vi "Close Session.vi"(8 "error in (no error)":errorcluster, 11 "VISA resource name":refnum<visa-resource-name>) -> ()   [LabVIEW 2014]
panel:
  in  "Reset? (T: Yes)":bool=TRUE
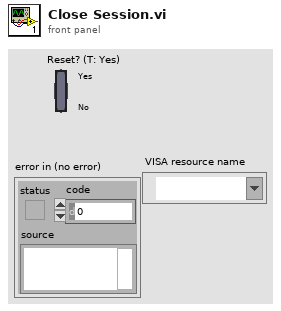
[diagram p1: front panel]
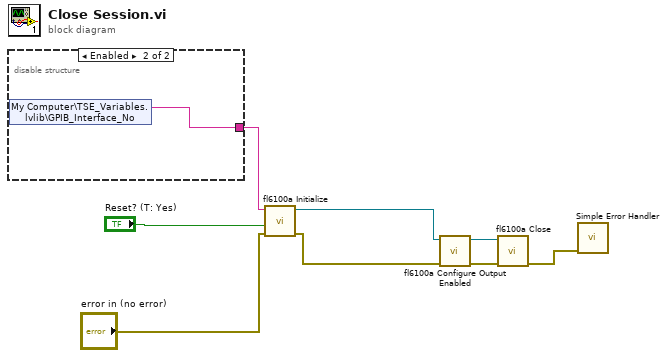
[diagram p0: block diagram]
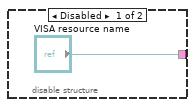
[diagram p2: hidden frame]
diagram:
  n1 = disable-structure shown="Enabled" {
    disable-tunnel: ["VISA resource name" w10] -> w4
    frame Disabled {
    }
    frame Enabled {
      n2 = shared-variable "My Computer\\TSE_Variables.lvlib\\GPIB_Interface_No"() -> (w10:string)  [unwired: 1 in, 1 out]
    }
  }
  n3 = call <instrlib>:"fl6100a Initialize.vi"("error in (no error)"="error in (no error)", "Reset? (T: Yes)"="Reset? (T: Yes)", "VISA resource name"=w4) -> ("error out"=w2:errorcluster, "VISA resource name out"=w1:refnum<visa-resource-name>)  [unwired: 7 in]
  n4 = call <instrlib>:"fl6100a Configure Output Enabled.vi"("error in (no error)"=w2, "VISA resource name"=w1) -> ("error out"=w6:errorcluster, "VISA resource name out"=w7:refnum<visa-resource-name>)  [unwired: 8 in]
  n5 = call <instrlib>:"fl6100a Close.vi"("error in (no error)"=w6, "VISA resource name"=w7) -> ("error out"=w8:errorcluster)  [unwired: 9 in]
  n6 = call <vilib>:"Simple Error Handler.vi"("error in (no error)"=w8) -> ()  [unwired: 4 in, 5 out]
